vi "NT Server Implementation.vi"(6 "Update Time":i32=100, 8 "error in (no error)":errorcluster, 9 "Timeout":i32=1000, 10 "Server Name":string, 11 "Enable Read Errors":bool) -> ()   [LabVIEW 2018]
doc: "This VI runs the Network Table services for the robot. It is intended to be run in parallel with the rest of the code. The top level of Robot Main is a good location. You may then read and write variables and they will be shared with Network Table clients."
uses:
  NT Globals.vi
  NI_LVConfig.lvlib
panel:
  in  "stop":bool
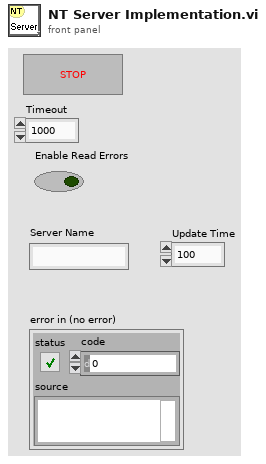
[diagram p1: front panel]
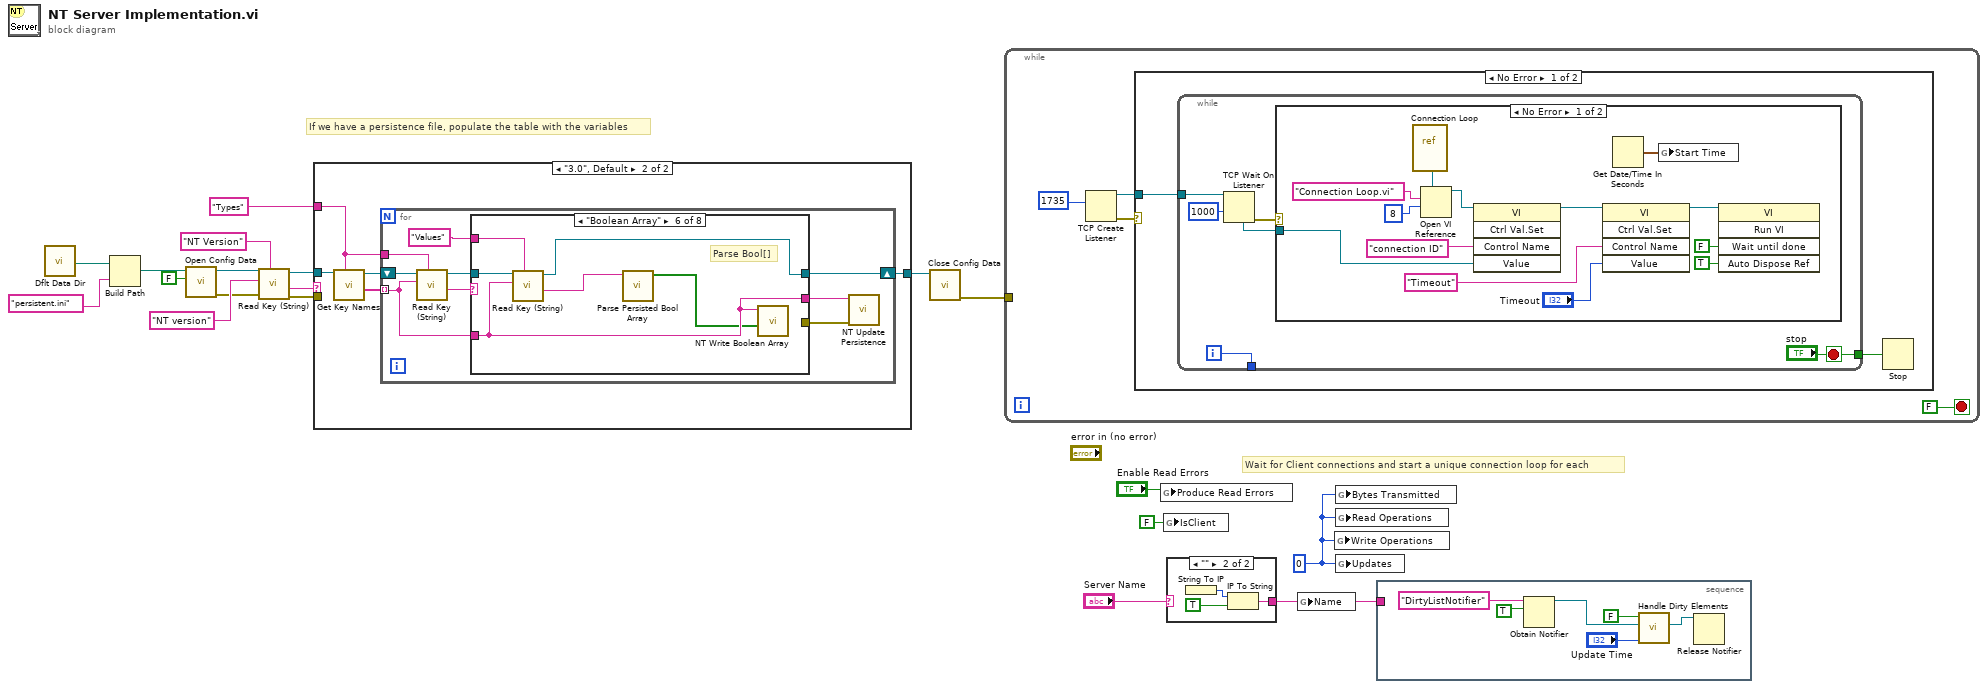
[diagram p0: block diagram]
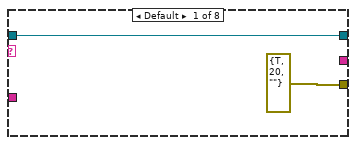
[diagram p3: hidden frame]
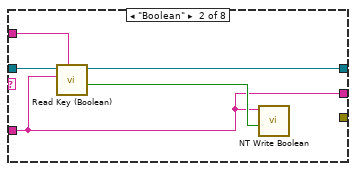
[diagram p4: hidden frame]
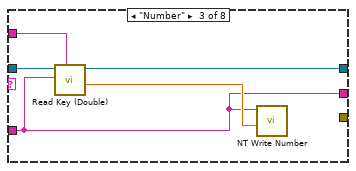
[diagram p5: hidden frame]
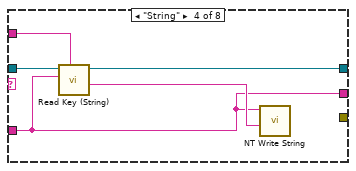
[diagram p6: hidden frame]
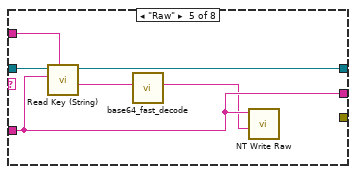
[diagram p7: hidden frame]
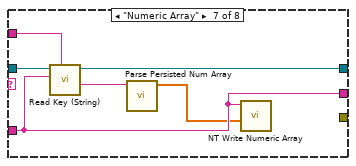
[diagram p8: hidden frame]
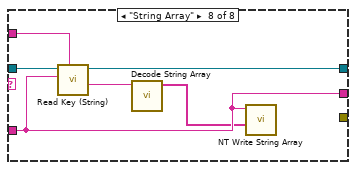
[diagram p9: hidden frame]
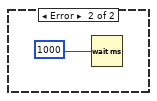
[diagram p10: hidden frame]
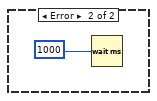
[diagram p11: hidden frame]
diagram:
  w17 = 0 ("Updates")
  # "If we have a persistence file, populate the table with the variables"
  # "Wait for Client connections and start a unique connection loop for each"
  n1 = call "Dflt Data Dir.vi"() -> ("App:Default Data Directory"=w13:path)
  n2 = Build Path(base path=w13, name or relative path="persistent.ini") -> (appended path=w4:path)
  n3 = call "Open Config Data.vi"("create file if necessary (T)"=FALSE, "configuration file path"=w4) -> ("error out"=w2:errorcluster, "refnum"=w6:refnum<k1>)  [unwired: 7 in, 1 out]
  n4 = call "Read Key (String).vi"("section"="NT Version", "error in (no error)"=w2, "key"="NT version" ("section"), "refnum"=w6) -> ("error out"=w1:errorcluster, "value"=w9:string, "refnum out"=w10:refnum<k1>)  [unwired: 4 in, 1 out]
  n5 = case shown="\"3.0\", Default" w9 {
    tunnel: w10 -> [w20 w25]
    tunnel: "Types" ("section") -> [_ w23]
    tunnel: [w20 w22] -> w12
    tunnel: w1 -> [_ _]
    frame "" {
    }
    frame "3.0", Default {
      n6 = call "Get Key Names.vi"("section"=w23, "refnum"=w25) -> ("key names"=w21:string[], "refnum out"=w24:refnum<k1>)  [unwired: 6 in, 2 out]
      n7 = for {
        tunnel: w21 -> [w28] mode=indexing
        shift-right: [w30] -> w22
        shift-left: w24 -> [w34]
        tunnel: w23 -> [w29]
        n8 = call "Read Key (String).vi"("section"=w29, "key"=w28, "refnum"=w34) -> ("value"=w33:string, "refnum out"=w32:refnum<k1>)  [unwired: 5 in, 2 out]
        n9 = case shown="\"Boolean Array\"" w33 {
          tunnel: w32 -> [w36 w41 w46 w51 w57 w63 w69 w75]
          tunnel: "Values" ("section") -> [_ w40 w43 w50 w55 w62 w67 w74]
          tunnel: [w36 w39 w45 w49 w56 w60 w68 w73] -> w30
          tunnel: w28 -> [_ w37 w42 w47 w54 w61 w66 w72]
          tunnel: [_ w37 w42 w47 w54 w61 w66 w72] -> w27
          tunnel: [errorcluster {"status"=TRUE, "code"=20, "source"=""} ("error in") _ _ _ _ _ _ _] -> w26
          frame Default {
          }
          frame "Boolean" {
            n10 = call "Read Key (Boolean).vi"("section"=w40, "key"=w37, "refnum"=w41) -> ("value"=w38:bool, "refnum out"=w39:refnum<k1>)  [unwired: 5 in, 2 out]
            n11 = call "NT Write Boolean.vi"("Boolean"=w38, "Name"=w37) -> ()  [unwired: 9 in, 1 out]
          }
          frame "Number" {
            n12 = call "Read Key (Double).vi"("section"=w43, "key"=w42, "refnum"=w46) -> ("value"=w44:dbl, "refnum out"=w45:refnum<k1>)  [unwired: 5 in, 2 out]
            n13 = call "NT Write Number.vi"("Numeric"=w44, "Name"=w42) -> ()  [unwired: 9 in, 1 out]
          }
          frame "String" {
            n14 = call "Read Key (String).vi"("section"=w50, "key"=w47, "refnum"=w51) -> ("value"=w48:string, "refnum out"=w49:refnum<k1>)  [unwired: 5 in, 2 out]
            n15 = call "NT Write String.vi"("String"=w48, "Name"=w47) -> ()  [unwired: 9 in, 1 out]
          }
          frame "Raw" {
            n16 = call "Read Key (String).vi"("section"=w55, "key"=w54, "refnum"=w57) -> ("value"=w53:string, "refnum out"=w56:refnum<k1>)  [unwired: 5 in, 2 out]
            n17 = call "base64_fast_decode.vi"("string in (base64-encoded)"=w53) -> ("string out (decoded)"=w52:string)  [unwired: 9 in, 1 out]
            n18 = call "NT Write Raw.vi"("Raw"=w52, "Name"=w54) -> ()  [unwired: 9 in, 1 out]
          }
          frame "Boolean Array" {
            # "Parse Bool[]"
            n19 = call "Read Key (String).vi"("section"=w62, "key"=w61, "refnum"=w63) -> ("value"=w59:string, "refnum out"=w60:refnum<k1>)  [unwired: 5 in, 2 out]
            n20 = call "Parse Persisted Bool Array.vi"("file string value"=w59) -> ("Array of Booleans"=w58:bool[])  [unwired: 9 in, 1 out]
            n21 = call "NT Write Boolean Array.vi"("Boolean Array"=w58, "Name"=w61) -> ()  [unwired: 9 in, 1 out]
          }
          frame "Numeric Array" {
            n22 = call "Read Key (String).vi"("section"=w67, "key"=w66, "refnum"=w69) -> ("value"=w65:string, "refnum out"=w68:refnum<k1>)  [unwired: 5 in, 2 out]
            n23 = call "Parse Persisted Num Array.vi"("file string value"=w65) -> ("Array of Booleans"=w64:dbl[])  [unwired: 9 in, 1 out]
            n24 = call "NT Write Numeric Array.vi"("Numeric Array"=w64, "Name"=w66) -> ()  [unwired: 9 in, 1 out]
          }
          frame "String Array" {
            n25 = call "Read Key (String).vi"("section"=w74, "key"=w72, "refnum"=w75) -> ("value"=w71:string, "refnum out"=w73:refnum<k1>)  [unwired: 5 in, 2 out]
            n26 = call "Decode String Array.vi"("Encoded String"=w71) -> ("Strings"=w70:string[])  [unwired: 10 in]
            n27 = call "NT Write String Array.vi"("String Array"=w70, "Name"=w72) -> ()  [unwired: 9 in, 1 out]
          }
        }
        n28 = call "NT Update Persistence.vi"("error in"=w26, "Name"=w27) -> ()  [unwired: 9 in, 1 out]
      }
    }
  }
  n29 = call "Close Config Data.vi"("refnum"=w12) -> ("error out"=w14:errorcluster)  [unwired: 9 in, 1 out]
  n30 = while {
    tunnel: w14 -> [_]
    stop <- FALSE stop-if-true
    n31 = TCP Create Listener(10:u16 1735 ("port")) -> (0:w77:errorcluster, 3:w78:refnum<k5>)  [unwired: 4 in, 1 out]
    n32 = case shown="No Error" w77 {
      tunnel: w78 -> [w81 _]
      frame No Error {
        n33 = while {
          tunnel: w81 -> [w87]
          tunnel: [w85] -> _
          tunnel: ["stop"] -> w80
          i -> [w85]
          stop <- "stop" stop-if-true
          n34 = TCP Wait On Listener(9:1000 ("timeout ms (wait forever: -1)"), 11:w87) -> (0:w84:errorcluster, 4:w86:refnum<k5>)  [unwired: 2 in, 3 out]
          n35 = case shown="No Error" w84 {
            tunnel: w86 -> [w99 _]
            frame No Error {
              n36 = vi-ref "Connection Loop.vi"() -> (w93:refnum<vi>)
              n37 = Open VI Reference(type specifier VI Refnum (for type only)=w93, vi path="Connection Loop.vi", options=8) -> (vi reference=w95:refnum<vi>)  [unwired: 3 in, 1 out]
              n38 = invoke class="VI" method="Ctrl Val.Set"(reference=w95, "Control Name"="connection ID", "Value"=w99) -> (reference out=w92:refnum<vi>)  [unwired: 2 in, 4 out]
              n39 = invoke class="VI" method="Ctrl Val.Set"(reference=w92, "Control Name"="Timeout", "Value"="Timeout") -> (reference out=w91:refnum<vi>)  [unwired: 2 in, 4 out]
              n40 = Get Date/Time In Seconds() -> (seconds since 1Jan1904=w100:timestamp)
              n41 = global write "NT Globals.vi" "Start Time"(w100) -> ()
              n42 = invoke class="VI" method="Run VI"(reference=w91, "Wait until done"=FALSE ("Wait Until Done"), "Auto Dispose Ref"=TRUE ("Auto Dispose Reference")) -> ()  [unwired: 2 in, 5 out]
            }
            frame Error {
              n43 = Wait (ms)(milliseconds to wait=1000 ("timeout ms (wait forever: -1)")) -> ()  [unwired: 1 out]
            }
          }
        }
        n44 = Stop(stop? (T)=w80) -> ()
      }
      frame Error {
        n45 = Wait (ms)(milliseconds to wait=1000 ("timeout ms (wait forever: -1)")) -> ()  [unwired: 1 out]
      }
    }
  }
  n46 = global write "NT Globals.vi" "Produce Read Errors"("Enable Read Errors") -> ()
  n47 = global write "NT Globals.vi" "IsClient"(FALSE ("IsClient")) -> ()
  n48 = case shown="\"\"" "Server Name" {
    selector: "Server Name" -> [w103 _]
    tunnel: [w103 w104] -> w15
    frame Default {
    }
    frame "" {
      n49 = String To IP() -> (0:w106:u32)  [unwired: 1 in]
      n50 = IP To String(1:TRUE ("dot notation? (F)"), 2:w106) -> (0:w104:string)
    }
  }
  n51 = global write "NT Globals.vi" "Name"(w15) -> ()
  n52 = global write "NT Globals.vi" "Write Operations"(w17) -> ()
  n53 = global write "NT Globals.vi" "Bytes Transmitted"(w17) -> ()
  n54 = global write "NT Globals.vi" "Read Operations"(w17) -> ()
  n55 = global write "NT Globals.vi" "Updates"(w17) -> ()
  n56 = stacked-sequence {
    tunnel: w15 -> [_]
    frame #0 {
      n57 = Obtain Notifier(name (unnamed)="DirtyListNotifier", notification data type=TRUE ("IsClient")) -> (notifier out=w108:refnum<notifier>)  [unwired: 2 in, 2 out]
      n58 = call "Handle Dirty Elements.vi"("Update Time"="Update Time", "notifier out"=w108, "IsClient"=FALSE) -> ("notifier out 2"=w107:refnum<notifier>)  [unwired: 8 in]
      n59 = Release Notifier(notifier=w107) -> ()  [unwired: 2 in, 3 out]
    }
  }
